vi "Execution Manager Async.vi"(8 "Reg Notifier":refnum<notifier>, 9 "Ready Handshake":refnum<notifier>, 10 "Reg Event":refnum<user-event>, 11 "Hierarchy":string) -> ()   [LabVIEW 2020, in "FlexBlocks.lvlib"]
uses:
  FlexBlocks.lvlib
  Block State.ctl
  Run Action.ctl
  Block Status.ctl
  Block Status with Error.ctl
  Command.ctl
  Worker Block.ctl
panel:
  in  "Close":bool
  in  "Step":bool
  in  "Run":bool
  out "Map":map{string, T1}(c390)
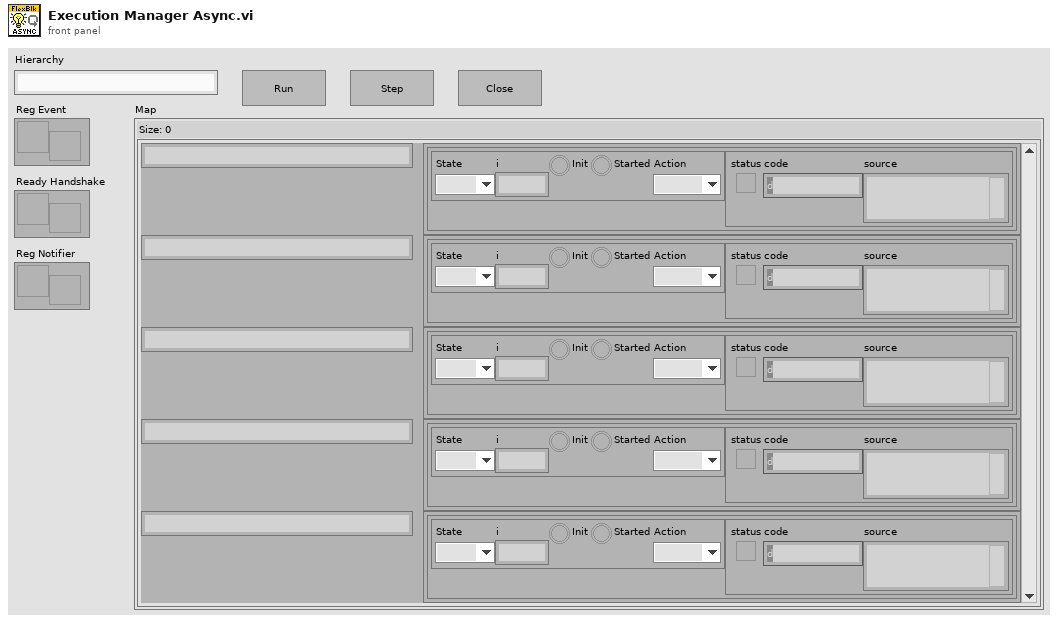
[diagram p1: front panel]
types:
  T1 = typedef "FlexBlocks.lvlib/Worker Block.ctl" = cluster{"Status Queue":refnum<queue>, "Command Queue":refnum<queue>, "Status":T2}
  T2 = typedef "FlexBlocks.lvlib/Block Status with Error.ctl" = cluster{"Status":T3, "Error":errorcluster}
  T3 = typedef "FlexBlocks.lvlib/Block Status.ctl" = cluster{"State":T4, "i":i32, "Init":bool, "Started":bool, "Action":T5}
  T4 = typedef "FlexBlocks.lvlib/Block State.ctl" = enum16{"Idle", "Init", "Start", "Run", "Stop"}
  T5 = typedef "FlexBlocks.lvlib/Run Action.ctl" = enum16{"N/A", "Read", "Work", "Write"}
  T6 = enum32{"Invalid", "Standard", "Closed", "Hidden", "Minimized", "Maximized"}
  T7 = typedef "FlexBlocks.lvlib/Command.ctl" = enum16{"Close", "Step", "Run", "Pause", "Init"}
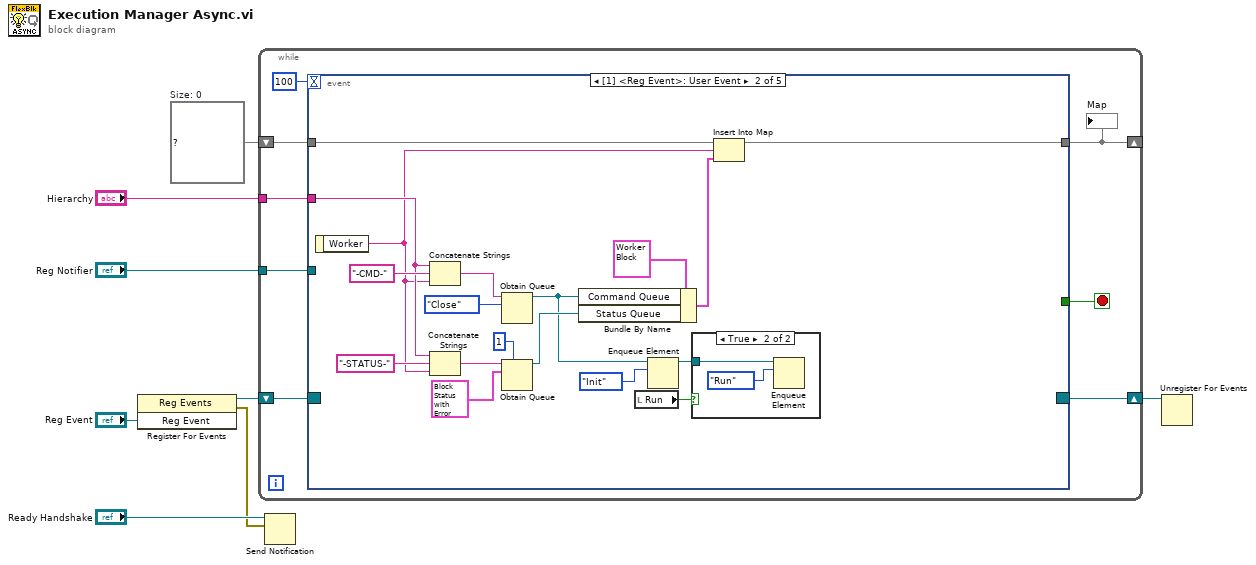
[diagram p0: block diagram]
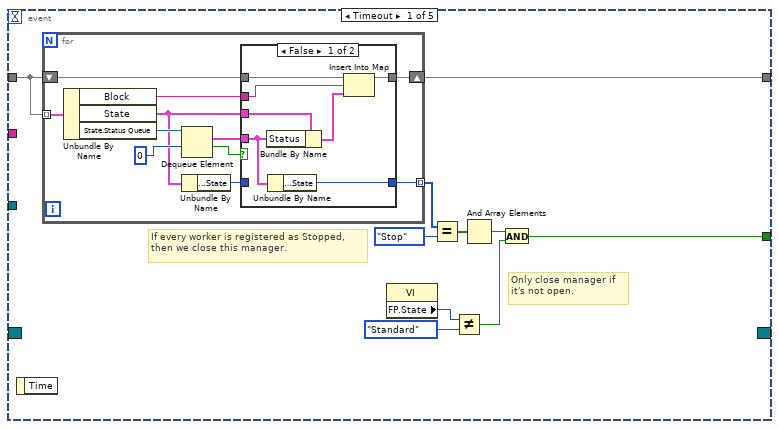
[diagram p2: hidden frame]
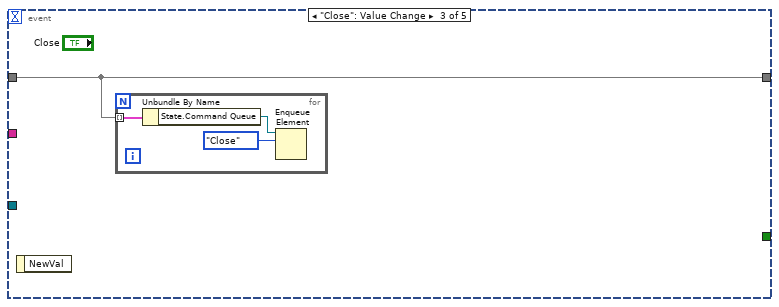
[diagram p5: hidden frame]
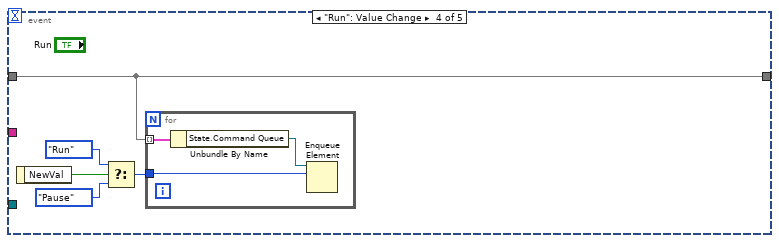
[diagram p6: hidden frame]
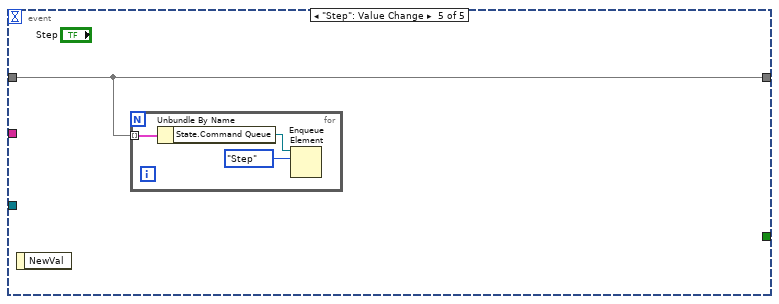
[diagram p7: hidden frame]
diagram:
  w2 = map{string, T1} {}  # Size: 0
  n1 = register-events("Reg Event") -> (reference out=w8:refnum<event-registration>, error out=w6:errorcluster)  [unwired: 2 in]
  n2 = while {
    shift-right: [w12] -> w3
    shift-left: w8 -> [w13]
    tunnel: "Hierarchy" -> [w14]
    tunnel: "Reg Notifier" -> [w15]
    shift-right: [w10] -> _
    shift-left: w2 -> [w11]
    stop <- w9 stop-if-true
    n3 = event shown="[1] <Reg Event>: User Event" {
      selector: w13 -> [_ _ _ _ _]
      dyn-events: [_ _ _ _ _] -> w12
      timeout: 100 -> [_ _ _ _ _]
      tunnel: w15 -> [_ _ _ _ _]
      tunnel: w14 -> [_ w57 _ _ _]
      tunnel: w11 -> [w26 w56 w67 w75 w79]
      tunnel: [w21 w51 w67 w75 w79] -> w10
      tunnel: [w18 _ _ _ _] -> w9
      event Timeout {
        # "Only close manager if it's not open."
        # "If every worker is registered as Stopped, then we close this manager."
        n4 = event-data() -> ()  [unwired: 1 in, 1 out]
        n5 = for {
          tunnel: w26 -> [w37] mode=indexing
          shift-right: [w31] -> w21
          shift-left: w26 -> [w34]
          tunnel: [w27] -> w25 mode=indexing
          n6 = Unbundle By Name(w37) -> ("Block"=w33:string, "State"=w29:T1, "State.Status Queue"=w36:refnum<queue>)
          n7 = Dequeue Element(queue=w36, timeout in ms (-1)=0) -> (element=w32:T2, timed out?=w30:bool)  [unwired: 1 in, 2 out]
          n8 = Unbundle By Name(w29) -> ("Status.Status.State"=w28:T4)
          n9 = case shown="False" w30 {
            tunnel: w34 -> [w43 w46]
            tunnel: w33 -> [w42 _]
            tunnel: w29 -> [w44 _]
            tunnel: w32 -> [w39 _]
            tunnel: [w40 w46] -> w31
            tunnel: w28 -> [_ w45]
            tunnel: [w38 w45] -> w27
            frame False {
              n10 = Bundle By Name(cluster=w44, "Status"=w39) -> (w41:T1)
              n11 = Unbundle By Name(w39) -> ("Status.State"=w38:T4)
              n12 = Insert Into Map(map in=w43, key=w42, value=w41) -> (map out=w40:map{string, T1})  [unwired: 2 out]
            }
            frame True {
            }
          }
        }
        n13 = property class="VI"() -> ("FP.State"=w20:T6)  [unwired: 2 in, 2 out]
        n14 = Equal?(x=w25, y=Block_State."Stop" ("Status.State")) -> (x = y?=w23:bool[])
        n15 = Not Equal?(x=w20, y=T6."Standard") -> (x != y?=w17:bool)
        n16 = And Array Elements(Boolean array=w23) -> (logical AND=w22:bool)
        n17 = And(x=w22, y=w17) -> (x .and. y?=w18:bool)
      }
      event User Event {
        n18 = event-data() -> ("Worker"=w52:string)  [unwired: 1 in]
        n19 = Concatenate Strings(w57, "-CMD-" ("string"), w52) -> (w64:string)
        n20 = Concatenate Strings(w57, "-STATUS-" ("string"), w52) -> (w62:string)
        n21 = Obtain Queue(name (unnamed)=w64, element data type=Command."Close" ("Command")) -> (queue out=w50:refnum<queue>)  [unwired: 3 in, 2 out]
        n22 = Obtain Queue(max queue size (-1, unlimited)=1, name (unnamed)=w62, element data type=T2 {"Status"={"State"=enum."Init", "i"=0, "Init"=FALSE, "Started"=FALSE, "Action"=enum."N/A"}, "Error"={"status"=FALSE, "code"=0, "source"=""}} ("Block Status with Error")) -> (queue out=w53:refnum<queue>)  [unwired: 2 in, 2 out]
        n23 = Bundle By Name(cluster=T1 {"Status Queue"=refnum, "Command Queue"=refnum, "Status"={"Status"={"State"=enum."Idle", "i"=0, "Init"=FALSE, "Started"=FALSE, "Action"=enum."N/A"}, "Error"={"status"=FALSE, "code"=0, "source"=""}}} ("value"), "Command Queue"=w50, "Status Queue"=w53) -> (w54:T1)
        n24 = local read "Run"() -> (w48:bool)
        n25 = Enqueue Element(queue=w50, element=Command."Init") -> (queue out=w47:refnum<queue>)  [unwired: 2 in, 2 out]
        n26 = case shown="True" w48 {
          tunnel: w47 -> [_ w66]
          frame False {
          }
          frame True {
            n27 = Enqueue Element(queue=w66, element=Command."Run") -> ()  [unwired: 2 in, 3 out]
          }
        }
        n28 = Insert Into Map(map in=w56, key=w52, value=w54) -> (map out=w51:map{string, T1})  [unwired: 2 out]
      }
      event "Close": Value Change {
        n29 = event-data() -> ()  [unwired: 1 in, 1 out]
        n30 = for {
          tunnel: w67 -> [w70] mode=indexing
          n31 = Unbundle By Name(w70) -> ("State.Command Queue"=w69:refnum<queue>)
          n32 = Enqueue Element(queue=w69, element=Command."Close") -> ()  [unwired: 2 in, 3 out]
        }
      }
      event "Run": Value Change {
        n33 = event-data() -> ("NewVal"=w74:bool)  [unwired: 1 in]
        n34 = Select(t=Command."Run" ("element"), s=w74, f=Command."Pause" ("element")) -> (s? t:f=w71:T7)
        n35 = for {
          tunnel: w75 -> [w78] mode=indexing
          tunnel: w71 -> [w76]
          n36 = Unbundle By Name(w78) -> ("State.Command Queue"=w77:refnum<queue>)
          n37 = Enqueue Element(queue=w77, element=w76) -> ()  [unwired: 2 in, 3 out]
        }
      }
      event "Step": Value Change {
        n38 = event-data() -> ()  [unwired: 1 in, 1 out]
        n39 = for {
          tunnel: w79 -> [w82] mode=indexing
          n40 = Unbundle By Name(w82) -> ("State.Command Queue"=w81:refnum<queue>)
          n41 = Enqueue Element(queue=w81, element=Command."Step") -> ()  [unwired: 2 in, 3 out]
        }
      }
    }
    "Map" <- w10
  }
  n42 = Send Notification(notification=w6, notifier="Ready Handshake") -> ()  [unwired: 1 in, 2 out]
  n43 = Unregister For Events(event registration refnum=w3) -> ()  [unwired: 1 in, 1 out]
